vi "GetLoopConditional.vi"(5 "Loop in":refnum<class "Loop.lvclass">, 6 "error in":errorcluster, 9 "VI Interpreter in":refnum<class "VI Interpreter.lvclass">) -> (0 "error out":errorcluster, 3 "VI Interpreter out":refnum<class "VI Interpreter.lvclass">, 4 "Loop out":refnum<class "Loop.lvclass">)   [LabVIEW 2014, in "Raspberry Pi Compatible Compiler for LabVIEW.lvlib" / "VI Interpreter.lvclass"]
uses:
  VI Interpreter.lvclass
  Loop/Loop.lvclass
  Loop/Loop.lvclass/Loop.ctl
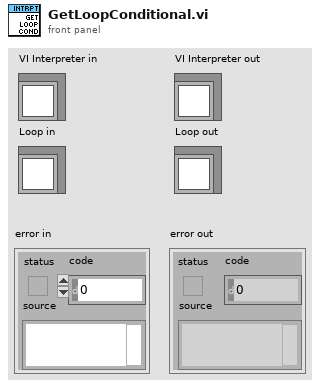
[diagram p1: front panel]
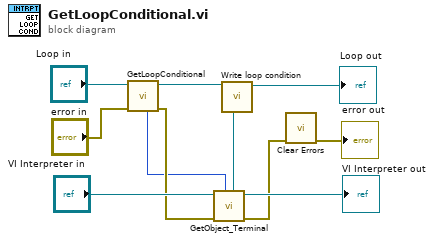
[diagram p0: block diagram]
diagram:
  n1 = call-dynamic "GetLoopConditional.vi"("error in"="error in", "Loop in"="Loop in") -> ("error out"=w5:errorcluster, "Loop out"=w6:refnum<class "Loop.lvclass">, "conditional UID"=w4:i32)  [unwired: 5 in]
  n2 = call "GetObject_Terminal.vi"("UID"=w4, "error in"=w5, "VI Interpreter in"="VI Interpreter in") -> ("error out"=w2:errorcluster, "VI Interpreter out"=→"VI Interpreter out":refnum<class "VI Interpreter.lvclass">, "Terminal"=w10:refnum<class "Terminal.lvclass">)  [unwired: 3 in, 1 out]
  n3 = call "Write loop condition.vi"("conditional terminal"=w10, "Loop in"=w6) -> ("Loop out"=→"Loop out":refnum<class "Loop.lvclass">)  [unwired: 7 in]
  n4 = call <vilib>:"Clear Errors.vi"("error in (no error)"=w2) -> ("error out"=→"error out":errorcluster)  [unwired: 5 in, 1 out]
